vi "CaculateBounds.vi"(7 "menu in":refnum<class "menu.lvclass">, 8 "error in (no error)":errorcluster, 11 "text in":refnum<class "text.lvclass">) -> (0 "error out":errorcluster, 2 "bounds":cluster{"width":u32, "height":u32}, 3 "text out":refnum<class "text.lvclass">)   [LabVIEW 2009, in "text.lvclass"]
uses:
  text.lvclass
  Menu/menu.lvclass
  text.lvclass/text.ctl
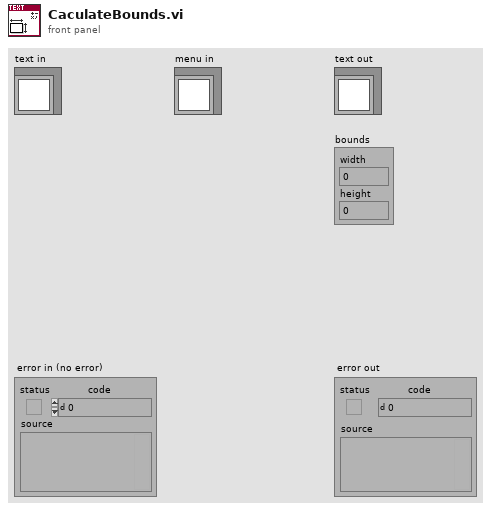
[diagram p1: front panel]
types:
  T1 = enum16{"Type?", "Plain", "Underline", "Parentheses", "End"}
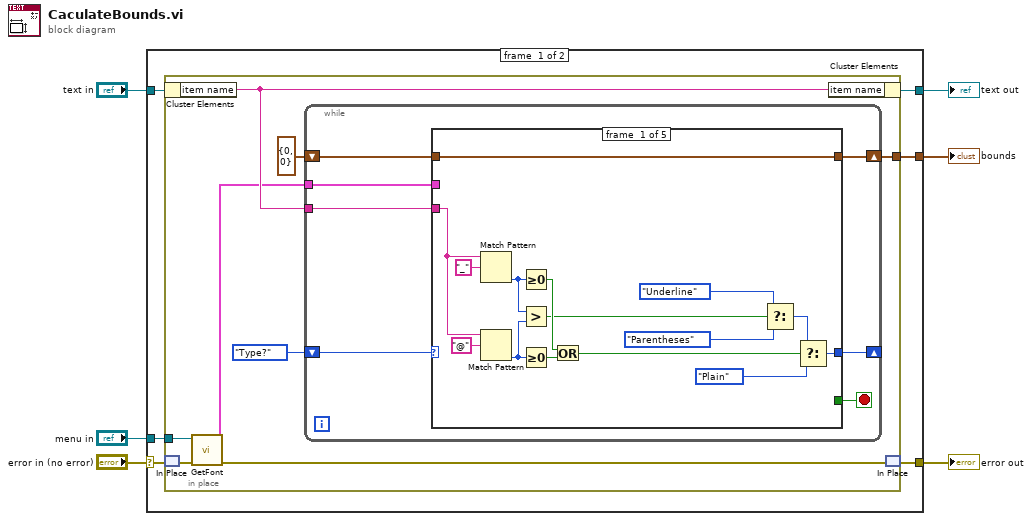
[diagram p0: block diagram]
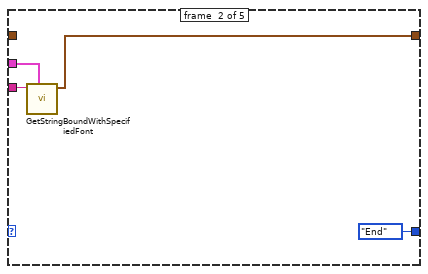
[diagram p2: hidden frame]
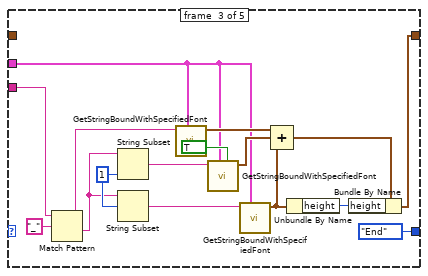
[diagram p3: hidden frame]
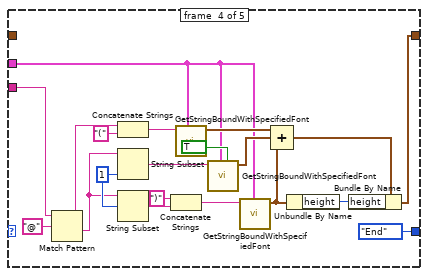
[diagram p4: hidden frame]
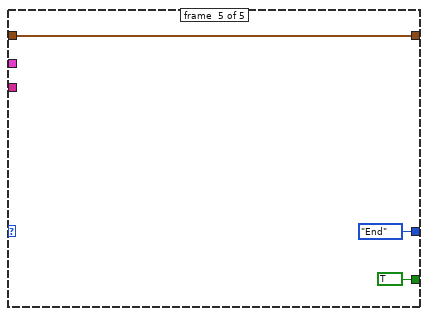
[diagram p5: hidden frame]
diagram:
  n1 = case shown="No Error" "error in (no error)" {
    selector: "error in (no error)" -> [w9 w87]
    tunnel: [w10 w87] -> w3
    tunnel: [w11 w86] -> w5
    tunnel: "text in" -> [w12 w86]
    tunnel: "menu in" -> [w8 _]
    tunnel: [w7 _] -> w1
    frame #0 {
      n2 = in-place {
        in-place-border: w8 -> [w17]
        in-place-border: [w13] -> w7
        n3 = in-place-cluster #1(w12) -> ("item name"=w19:string)
        n4 = in-place-match #2(w9) -> (w16:errorcluster)
        n5 = call "GetFont.vi"("error in (no error)"=w16, "menu in"=w17) -> ("error out"=w15:errorcluster, "font"=w14:cluster{"name":string, "size":i16, "color":u32})  [unwired: 7 in, 1 out]
        n6 = while {
          shift-right: [w26] -> _
          shift-left: T1."Type?" ("state") -> [w27]
          tunnel: w19 -> [w25]
          shift-right: [w23] -> w13
          shift-left: cluster{"width":u32, "height":u32} {"width"=0, "height"=0} ("bounds") -> [w24]
          tunnel: w14 -> [w21]
          stop <- w22 stop-if-true
          n7 = case shown="\"Type?\"" w27 {
            tunnel: [w41 T1."End" ("state") T1."End" ("state") T1."End" ("state") T1."End" ("state")] -> w26
            tunnel: w25 -> [w36 w46 w59 w75 _]
            tunnel: w24 -> [w40 _ _ _ w85]
            tunnel: [w40 w45 w49 w63 w85] -> w23
            tunnel: [_ _ _ _ TRUE] -> w22
            tunnel: w21 -> [_ w43 w50 w67 _]
            frame #0 {
              n8 = Match Pattern(string=w36, regular expression="_") -> (offset past match=w29:i32)  [unwired: 1 in, 3 out]
              n9 = Match Pattern(string=w36, regular expression="@") -> (offset past match=w28:i32)  [unwired: 1 in, 3 out]
              n10 = Greater Or Equal To 0?(x=w29) -> (x >= 0?=w33:bool)
              n11 = Greater?(x=w29, y=w28) -> (0:w30:bool)
              n12 = Greater Or Equal To 0?(x=w28) -> (x >= 0?=w34:bool)
              n13 = Or(x=w33, y=w34) -> (x .or. y?=w35:bool)
              n14 = Select(t=T1."Underline" ("state"), s=w30, f=T1."Parentheses" ("state")) -> (s? t:f=w37:T1)
              n15 = Select(t=w37, s=w35, f=T1."Plain" ("state")) -> (s? t:f=w41:T1)
            }
            frame #1 {
              n16 = call "GetStringBoundWithSpecifiedFont.vi"("string"=w46, "font"=w43) -> ("bounds"=w45:cluster{"width":u32, "height":u32})  [unwired: 9 in]
            }
            frame #2 {
              w61 = 1 ("length (rest)")
              n17 = Match Pattern(string=w59, regular expression="_") -> (before substring=w52:string, after substring=w60:string)  [unwired: 1 in, 2 out]
              n18 = String Subset(string=w60, length (rest)=w61) -> (substring=w58:string)  [unwired: 1 in]
              n19 = String Subset(string=w60, offset (0)=w61) -> (substring=w53:string)  [unwired: 1 in]
              n20 = call "GetStringBoundWithSpecifiedFont.vi"("string"=w52, "font"=w50) -> ("bounds"=w56:cluster{"width":u32, "height":u32})  [unwired: 9 in]
              n21 = call "GetStringBoundWithSpecifiedFont.vi"("string"=w58, "font"=w50, "underline? (F)"=TRUE) -> ("bounds"=w55:cluster{"width":u32, "height":u32})  [unwired: 8 in]
              n22 = call "GetStringBoundWithSpecifiedFont.vi"("string"=w53, "font"=w50) -> ("bounds"=w48:cluster{"width":u32, "height":u32})  [unwired: 9 in]
              n23 = Compound Arithmetic op=ADD(w56, w55, w48) -> (w54:cluster{"width":u32, "height":u32})
              n24 = Unbundle By Name(w48) -> ("height"=w47:u32)
              n25 = Bundle By Name(cluster=w54, "height"=w47) -> (w49:cluster{"width":u32, "height":u32})
            }
            frame #3 {
              w81 = 1 ("length (rest)")
              n26 = Match Pattern(string=w75, regular expression="@") -> (before substring=w78:string, after substring=w79:string)  [unwired: 1 in, 2 out]
              n27 = Concatenate Strings(w78, "(" ("string")) -> (w74:string)
              n28 = String Subset(string=w79, length (rest)=w81) -> (substring=w73:string)  [unwired: 1 in]
              n29 = String Subset(string=w79, offset (0)=w81) -> (substring=w80:string)  [unwired: 1 in]
              n30 = Concatenate Strings(")" ("string"), w80) -> (w72:string)
              n31 = call "GetStringBoundWithSpecifiedFont.vi"("string"=w74, "font"=w67) -> ("bounds"=w70:cluster{"width":u32, "height":u32})  [unwired: 9 in]
              n32 = call "GetStringBoundWithSpecifiedFont.vi"("string"=w73, "font"=w67, "underline? (F)"=TRUE) -> ("bounds"=w69:cluster{"width":u32, "height":u32})  [unwired: 8 in]
              n33 = call "GetStringBoundWithSpecifiedFont.vi"("string"=w72, "font"=w67) -> ("bounds"=w65:cluster{"width":u32, "height":u32})  [unwired: 9 in]
              n34 = Compound Arithmetic op=ADD(w70, w69, w65) -> (w64:cluster{"width":u32, "height":u32})
              n35 = Unbundle By Name(w65) -> ("height"=w66:u32)
              n36 = Bundle By Name(cluster=w64, "height"=w66) -> (w63:cluster{"width":u32, "height":u32})
            }
            frame #4 {
            }
          }
        }
        n37 = in-place-cluster #1("item name"=w19) -> (w11:refnum<class "text.lvclass">)
        n38 = in-place-match #2(w15) -> (w10:errorcluster)
      }
    }
    frame #1 {
    }
  }
  "text out" <- w5
  "error out" <- w3
  "bounds" <- w1
